vi "Create Instance Impl.vi"(8 "error in (no error)":errorcluster, 10 "Stage Configuration":T1={"Serial Port"="COM4", "Forward Step (mm)"=0.4, "Lane Length (mm)"=6.0, "Lane Separation (mm)"=0.8, "Stage Type"=enum."Ti2", "Autofocus Z Planes"=9, "Autofocus Range (um)"=30.0, "Stage Limits"={"Y Min"=-4.5, "Y Max"=3.0, "X Min"=-19.0, "X Max"=33.5}, "Slide (mm)"={"top"=-13.0, "right"=-22.3, "width"=60.0, "height"=25.4}}, 11 "Ludl Stage in":refnum<class "Ludl Stage.lvclass">) -> (0 "error out":errorcluster, 3 "Ludl Stage out":refnum<class "Ludl Stage.lvclass">)   [LabVIEW 2023, in "Ludl Stage.lvlib" / "Ludl Stage.lvclass"]
uses:
  Ludl Stage.lvclass
  Resources/Type Defs/Stage Configuration.ctl
  <vilib>/Instr/_visa.llb/VISA Configure Serial Port (Instr).vi
  Ludl Stage.lvclass/Ludl Stage.ctl
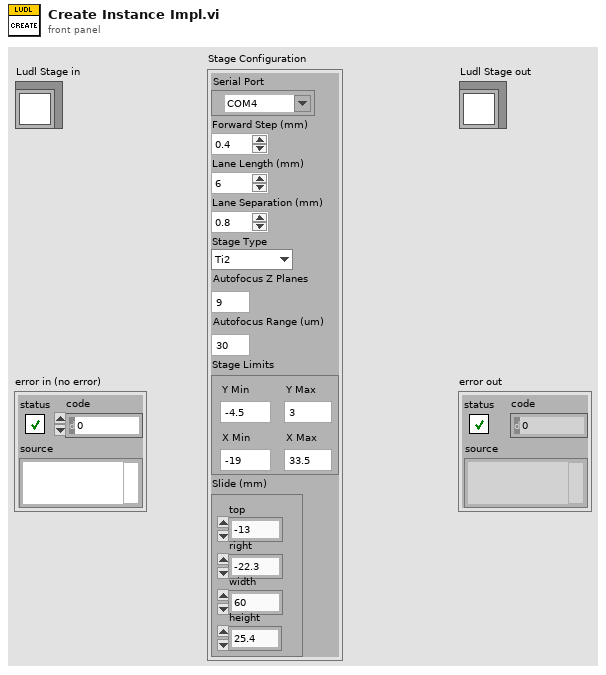
[diagram p1: front panel]
types:
  T1 = typedef "Stage Configuration.ctl" = cluster{"Serial Port":refnum<visa-resource-name>, "Forward Step (mm)":dbl, "Lane Length (mm)":dbl, "Lane Separation (mm)":dbl, "Stage Type":enum16{"Disabled", "ESP301", "Ti2", "Ludl", "ASI"}, "Autofocus Z Planes":i32, "Autofocus Range (um)":dbl, "Stage Limits":cluster{"Y Min":dbl, "Y Max":dbl, "X Min":dbl, "X Max":dbl}, "Slide (mm)":cluster{"top":dbl, "right":dbl, "width":dbl, "height":dbl}}
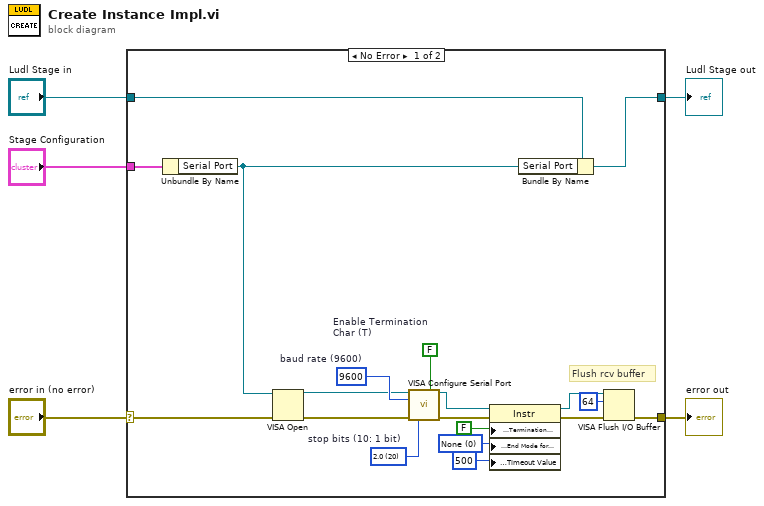
[diagram p0: block diagram]
diagram:
  n1 = case shown="No Error" "error in (no error)" {
    selector: "error in (no error)" -> [w11 w25]
    tunnel: [w10 w25] -> w4
    tunnel: "Ludl Stage in" -> [w8 w26]
    tunnel: [w7 w26] -> w2
    tunnel: "Stage Configuration" -> [w9 _]
    frame No Error {
      w17 = u16 0 items=["None", "LastBit", "TermChar"] ("Serial Settings:Serial End Mode for Reads")
      w22 = u16 20 items=["1.0"=10, "1.5"=15, "2.0"=20]  # stop bits (10: 1 bit)
      w24 = FALSE  # Enable Termination Char (T)
      w23 = u32 9600  # baud rate (9600)
      # "Flush rcv buffer"
      n2 = Unbundle By Name(w9) -> ("Serial Port"=w6:refnum<visa-resource-name>)
      n3 = VISA Open(error in (no error)=w11, VISA resource name=w6) -> (VISA resource name=w20:refnum<visa-resource-name>, error out=w21:errorcluster)  [unwired: 3 in]
      n4 = call-poly "VISA Configure Serial Port"("VISA resource name"=w20, "Enable Termination\nChar (T)"=w24, "baud rate (9600)"=w23, "error in (no error)"=w21, "stop bits (10: 1 bit)"=w22) -> ("VISA resource name out"=w15:refnum<visa-resource-name>, "error out"=w12:errorcluster)  [unwired: 9 in]
      n5 = property class="Instr"(reference=w15, error in=w12, "Message Based Settings:Termination Character Enable"=FALSE, "Serial Settings:End Mode for Reads"=w17, "General Settings:Timeout Value"=u32 500) -> (reference out=w14:refnum<visa-resource-name>, error out=w13:errorcluster)
      n6 = Bundle By Name(cluster=w8, "Serial Port"=w6) -> (w7:refnum<class "Ludl Stage.lvclass">)
      n7 = VISA Flush I/O Buffer(VISA resource name=w14, mask (16)=u16 64, error in (no error)=w13) -> (error out=w10:errorcluster)  [unwired: 1 out]
    }
    frame Error {
    }
  }
  "error out" <- w4
  "Ludl Stage out" <- w2
